vi "RT Loop - Propotional Update.vi"(11 "Message Queue":refnum<queue>) -> ()   [LabVIEW 2018]
doc: "This Control Loop VI performs control calculations of diverter line (DL) rotation."
uses:
  Support/Message Queue/Message Cluster.ctl
  Support/Message Queue/Message.ctl
  <vilib>/Platform/TimedLoop/XDataNode/timing_clust.ctl
  <vilib>/Platform/TimedLoop/XDataNode/nitl_modes.ctl
  <vilib>/Platform/TimedLoop/XDataNode/wakeup.ctl
  Controls/Propotional State.ctl
  <vilib>/Platform/TimedLoop/XDataNode/loadnilvce.vi
  Globals/Global - RT Channels.vi
  Globals/Global - Parameters.vi
  <vilib>/Platform/TimedLoop/XDataNode/XDataNode.xnode
  <vilib>/Platform/TimedLoop/XDataNode/XDNodeRunTimeDep.lvlib
  support/Message Queue/Message Queue.lvlib
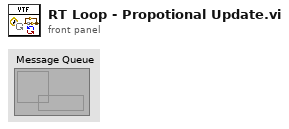
[diagram p1: front panel]
types:
  T1 = typedef "XDNodeRunTimeDep.lvlib/timing_clust.ctl" = cluster{"Expected End [f-1]":u64, "Actual End [f-1]":u64, "Finished Late? [f-1]":bool, "Expected End [i-1]":u64, "Actual End [i-1]":u64, "Finished Late? [i-1]":bool, "Expected Start [i]":u64, "Actual Start [i]":u64, "Expected Start [f]":u64, "Actual Start [f]":u64, "Source Name":string, "Structure Name":string, "Period":i64, "Deadline":i64, "Offset":i64, "Start":i64, "Priority":i32, "Timeout":i32, "Mode":T2, "Wakeup Reason":T3, "Error":errorcluster, "Source Type":string, "Secondary Source Type":string, "Global End Time":u64, "Global Start Time":u64, "Frame Duration":u64, "Iteration Duration":u64, "Assigned CPU":i32, "I/O Scan Engine Mode":u32}
  T2 = typedef "XDNodeRunTimeDep.lvlib/nitl_modes.ctl" = enum32{"No Change", "Process missed periods, maintain original phase", "Discard missed periods, maintain original phase", "Process missed periods, ignore original phase", "Discard missed periods, ignore original phase"}
  T3 = typedef "XDNodeRunTimeDep.lvlib/wakeup.ctl" = enum32{"Normal", "Aborted", "Asynchronous wakeup", "Timing source error", "Timed loop error", "Timeout"}
  T4 = typedef "Propotional State.ctl" = enum16{"Initilize All", "Do Nothing", "AB Valve Update", "TC Valve Update", "Bleed Valve Update", "Triplex Pump Update"}
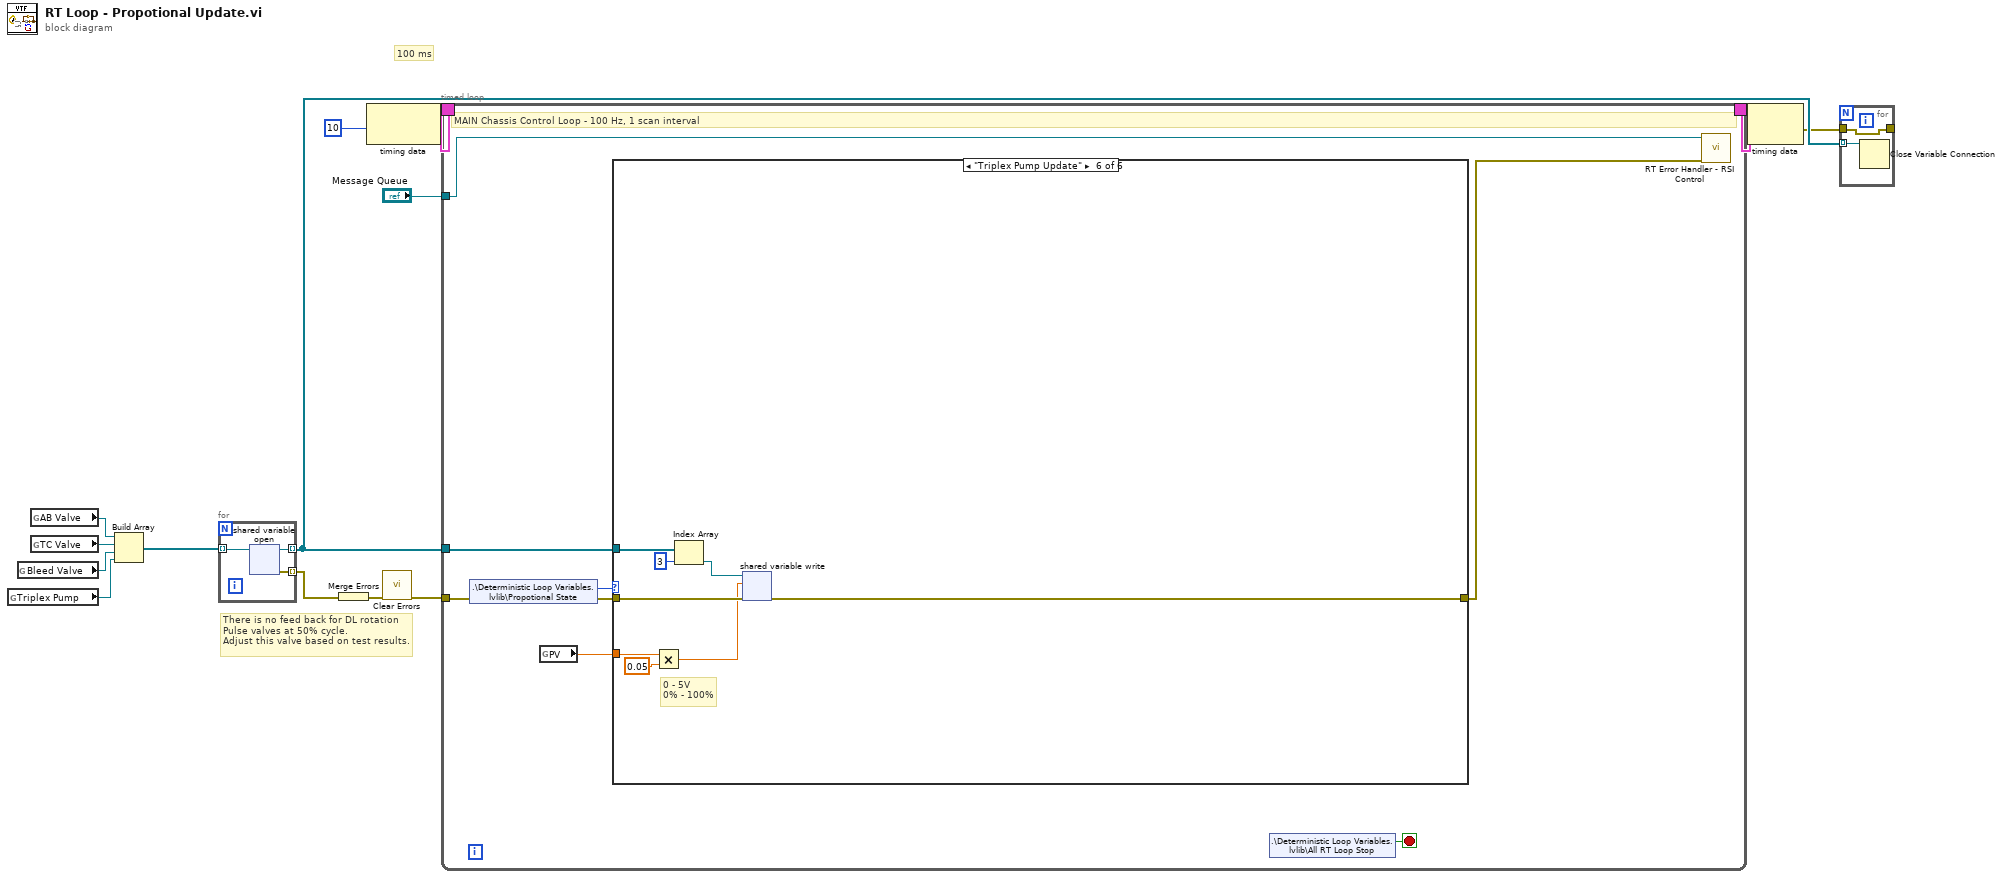
[diagram p0: block diagram]
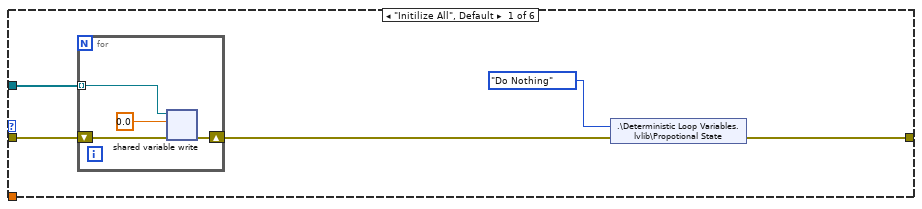
[diagram p2: hidden frame]
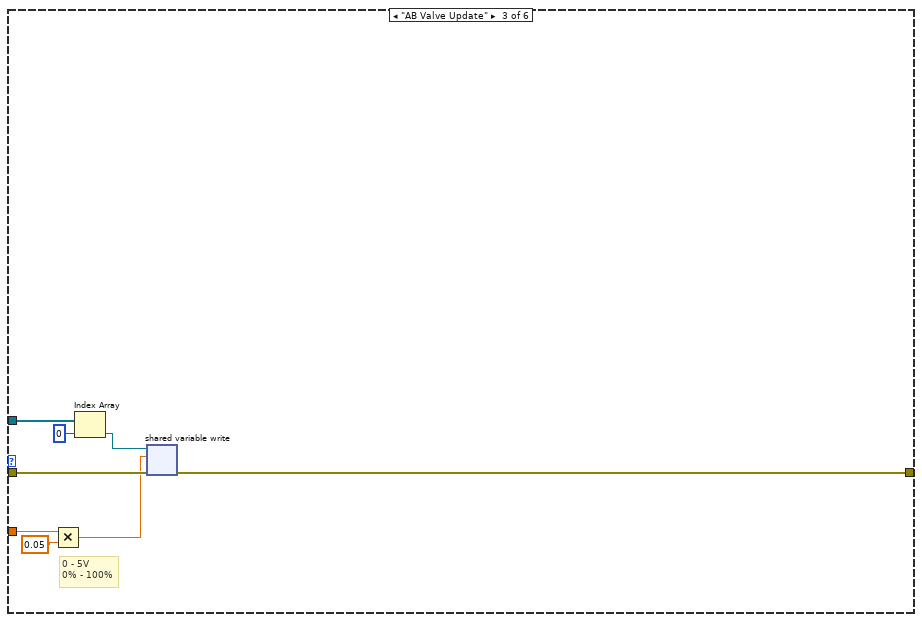
[diagram p4: hidden frame]
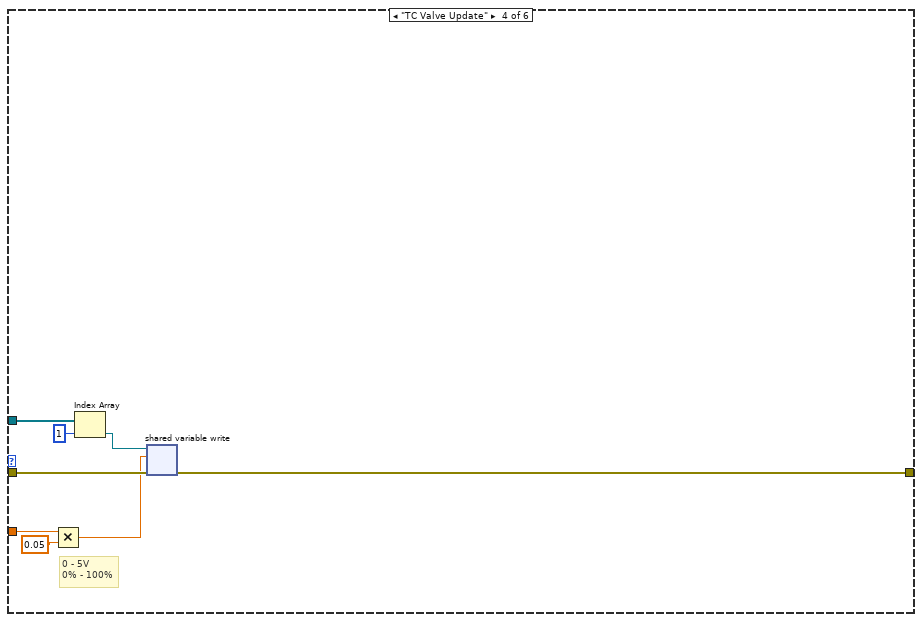
[diagram p5: hidden frame]
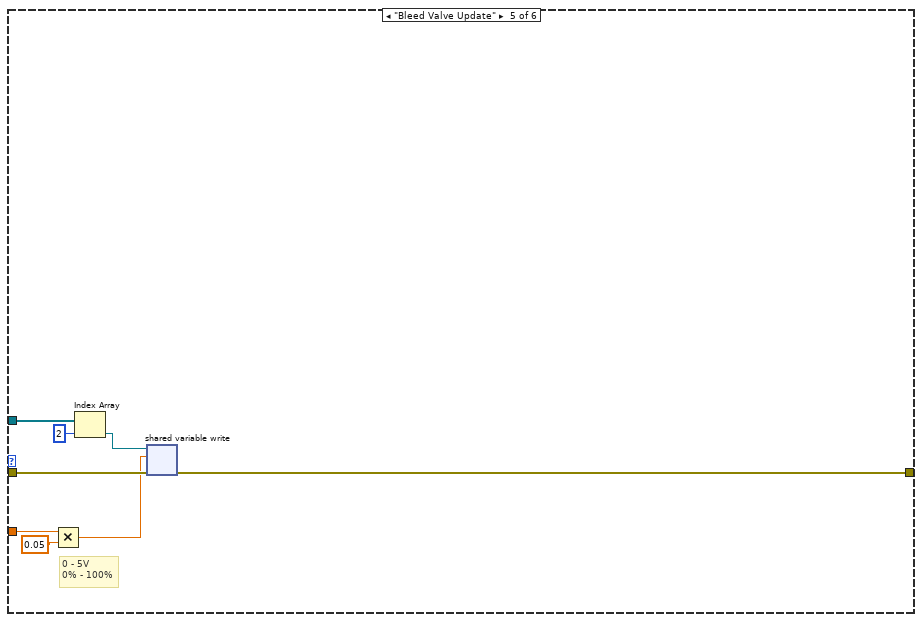
[diagram p6: hidden frame]
diagram:
  # "100 ms"
  # "There is no feed back for DL rotation\nPulse valves at 50% cycle. \nAdjust this valve based on test results."
  n1 = global read "Global - RT Channels.vi" "Triplex Pump"() -> (w3:refnum<k21>)
  n2 = global read "Global - RT Channels.vi" "Bleed Valve"() -> (w4:refnum<k21>)
  n3 = global read "Global - RT Channels.vi" "AB Valve"() -> (w2:refnum<k21>)
  n4 = global read "Global - RT Channels.vi" "TC Valve"() -> (w1:refnum<k21>)
  n5 = Build Array(w2, w1, w4, w3) -> (w5:refnum<k21>[])
  n6 = for {
    tunnel: w5 -> [w15] mode=indexing
    tunnel: [w17] -> w9 mode=indexing
    tunnel: [w16] -> w6 mode=indexing
    n7 = shared-variable-open(w15) -> (w17:refnum<k21>, w16:errorcluster)  [unwired: 1 in]
  }
  n8 = Merge Errors(w6) -> (w7:errorcluster)
  n9 = node-c288(i64 10 ("Period")) -> (w14:T1)
  n10 = call <vilib>:"Clear Errors.vi"("error in (no error)"=w7) -> ("error out"=w10:errorcluster)  [unwired: 5 in, 1 out]
  n11 = timed-loop {
    timing: w14 -> [_]
    timing-out: [_] -> w13
    tunnel: "Message Queue" -> [w24]
    tunnel: w10 -> [w22]
    tunnel: w9 -> [w19]
    stop <- w25 stop-if-true
    # "MAIN Chassis Control Loop - 100 Hz, 1 scan interval"
    n12 = shared-variable ".\\Deterministic Loop Variables.lvlib\\Propotional State"(error in=w22) -> (w20:T4, error out=w21:errorcluster)
    n13 = global read "Global - Parameters.vi" "PV"() -> (w18:dbl)
    n14 = case shown="\"Triplex Pump Update\"" w20 {
      tunnel: [w30 w35 w42 w50 w58 w66] -> w23
      tunnel: w21 -> [w27 w35 w43 w51 w59 w67]
      tunnel: w19 -> [w28 _ w38 w46 w54 w62]
      tunnel: w18 -> [_ _ w41 w49 w57 w65]
      frame "Initilize All", Default {
        n15 = for {
          tunnel: w28 -> [w32] mode=indexing
          shift-right: [w33] -> w26
          shift-left: w27 -> [w34]
          n16 = shared-variable-write(w32, w34, 0.0 ("data in")) -> (w33:errorcluster)  [unwired: 1 out]
        }
        n17 = shared-variable ".\\Deterministic Loop Variables.lvlib\\Propotional State"(Propotional_State."Do Nothing" ("Propotional State"), error in=w26) -> (error out=w30:errorcluster)
      }
      frame "Do Nothing" {
      }
      frame "AB Valve Update" {
        # "0 - 5V \n0% - 100%"
        n18 = Multiply(x=w41, y=0.05) -> (x*y=w39:dbl)
        n19 = Index Array(array=w38, index=0) -> (element=w36:refnum<k21>)
        n20 = shared-variable-write(w36, w43, w39) -> (w42:errorcluster)  [unwired: 1 out]
      }
      frame "TC Valve Update" {
        # "0 - 5V \n0% - 100%"
        n21 = Multiply(x=w49, y=0.05) -> (x*y=w47:dbl)
        n22 = Index Array(array=w46, index=1) -> (element=w44:refnum<k21>)
        n23 = shared-variable-write(w44, w51, w47) -> (w50:errorcluster)  [unwired: 1 out]
      }
      frame "Bleed Valve Update" {
        # "0 - 5V \n0% - 100%"
        n24 = Multiply(x=w57, y=0.05) -> (x*y=w55:dbl)
        n25 = Index Array(array=w54, index=2) -> (element=w52:refnum<k21>)
        n26 = shared-variable-write(w52, w59, w55) -> (w58:errorcluster)  [unwired: 1 out]
      }
      frame "Triplex Pump Update" {
        # "0 - 5V \n0% - 100%"
        n27 = Multiply(x=w65, y=0.05) -> (x*y=w63:dbl)
        n28 = Index Array(array=w62, index=3) -> (element=w60:refnum<k21>)
        n29 = shared-variable-write(w60, w67, w63) -> (w66:errorcluster)  [unwired: 1 out]
      }
    }
    n30 = shared-variable ".\\Deterministic Loop Variables.lvlib\\All RT Loop Stop"() -> (w25:bool)  [unwired: 1 in, 1 out]
    n31 = call "RT Error Handler - RSI Control.vi"("error in (no error)"=w23, "Message Queue"=w24) -> ()  [unwired: 8 in, 2 out]
  }
  n32 = node-c288(w13) -> (w8:errorcluster)
  n33 = for {
    tunnel: w8 -> [w70]
    tunnel: w9 -> [w71] mode=indexing
    tunnel: [w70] -> _
    n34 = Close Variable Connection(11:w71) -> ()  [unwired: 1 in, 1 out]
  }
